vi "Motion_Read Loader Discretes.vi"(8 "error in (no error)":errorcluster, 11 "TCP Connection Refnum in":refnum<k5>) -> (0 "error out":errorcluster, 2 "Loader Discretes":T1, 3 "TCP Connection Refnum (dup)":refnum<k5>)   [LabVIEW 2010]
uses:
  <vilib>/NI Modbus.llb/MB Ethernet Master Query Read Discrete Inputs (poly).vi
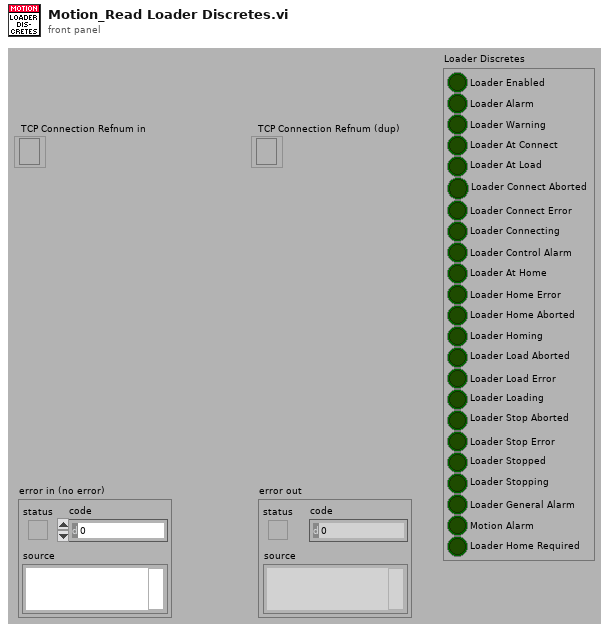
[diagram p1: front panel]
types:
  T1 = cluster{"Loader Enabled":bool, "Loader Alarm ":bool, "Loader Warning":bool, "Loader At Connect":bool, "Loader At Load":bool, "Loader Connect Aborted":bool, "Loader Connect Error":bool, "Loader Connecting":bool, "Loader Control Alarm":bool, "Loader At Home":bool, "Loader Home Error":bool, "Loader Home Aborted":bool, "Loader Homing":bool, "Loader Load Aborted":bool, "Loader Load Error":bool, "Loader Loading":bool, "Loader Stop Aborted":bool, "Loader Stop Error":bool, "Loader Stopped":bool, "Loader Stopping":bool, "Loader General Alarm":bool, "Motion Alarm":bool, "Loader Home Required":bool}
  T2 = cluster{"[0]":bool, "[1]":bool, "[2]":bool, "[3]":bool, "[4]":bool, "[5]":bool, "[6]":bool, "[7]":bool, "[8]":bool, "[9]":bool, "[10]":bool, "[11]":bool, "[12]":bool, "[13]":bool, "[14]":bool, "[15]":bool, "[16]":bool, "[17]":bool, "[18]":bool, "[19]":bool, "[20]":bool, "[21]":bool, "[22]":bool}
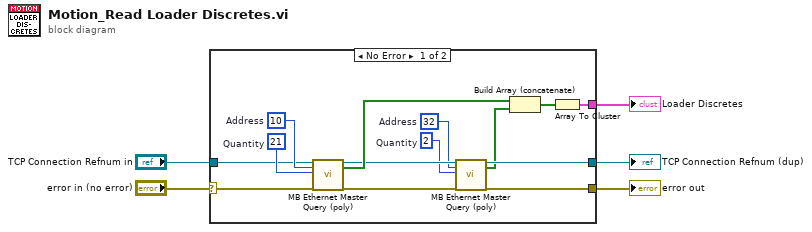
[diagram p0: block diagram]
diagram:
  n1 = case shown="No Error" "error in (no error)" {
    selector: "error in (no error)" -> [w16 w20]
    tunnel: [w17 _] -> w1
    tunnel: [w9 w20] -> w4
    tunnel: [w10 w21] -> w3
    tunnel: "TCP Connection Refnum in" -> [w15 w21]
    frame No Error {
      w7 = u16 2  # Quantity
      w8 = u16 32  # Address
      w18 = u16 21  # Quantity
      w19 = u16 10  # Address
      n2 = call-poly <vilib>:"MB Ethernet Master Query (poly).vi"("TCP Connection Refnum in"=w15, "Starting Address"=w19, "Quantity"=w18, "error in"=w16) -> ("TCP Connection Refnum (dup)"=w11:refnum<k5>, "Discrete Inputs"=w14:bool[], "error out"=w12:errorcluster)  [unwired: 12 in, 1 out]
      n3 = call-poly <vilib>:"MB Ethernet Master Query (poly).vi"("TCP Connection Refnum in"=w11, "Starting Address"=w8, "Quantity"=w7, "error in"=w12) -> ("TCP Connection Refnum (dup)"=w10:refnum<k5>, "Discrete Inputs"=w6:bool[], "error out"=w9:errorcluster)  [unwired: 12 in, 1 out]
      n4 = Build Array (concatenate)(w14, w6) -> (w13:bool[])
      n5 = Array To Cluster(array=w13) -> (cluster=w17:T2)
    }
    frame Error {
    }
  }
  "Loader Discretes" <- w1
  "error out" <- w4
  "TCP Connection Refnum (dup)" <- w3
